vi "Configure Timebase Mode.vi"(6 "Window Range (5.0E-6)":dbl=5e-06, 8 "error in (no error)":errorcluster, 9 "Window Position (0.0 s)":dbl, 10 "Timebase Mode (0: Main)":u16(ring) items=["Main", "Window", "XY", "Roll"], 11 "VISA resource name":refnum<visa-resource-name>) -> (0 "error out":errorcluster, 3 "VISA resource name out":refnum<visa-resource-name>)   [LabVIEW 2017, in "Agilent 6000 Series.lvlib"]
doc: "This VI selects time base mode.\n\n<B>NOTE:</B>\n\nThe Window Timebase and Window Range controls are only valid when Timebase Mode is set to \"Window\"."
uses:
  <instrlib>/Agilent 6000 Series/Agilent 6000 Series.lvlib
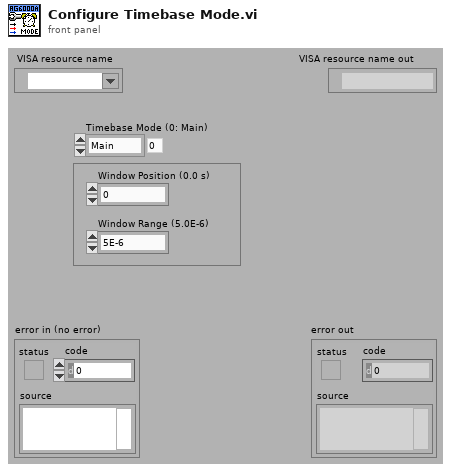
[diagram p1: front panel]
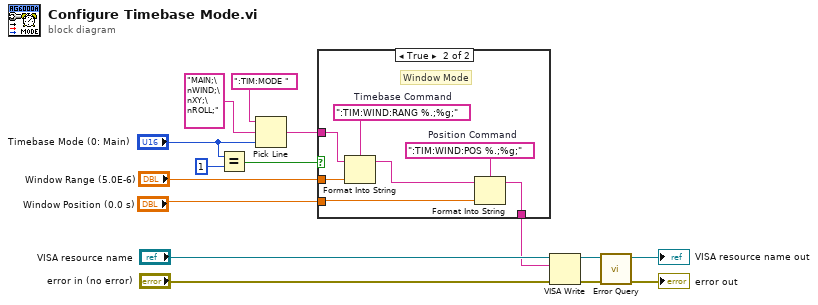
[diagram p0: block diagram]
diagram:
  n1 = Equal?(x="Timebase Mode (0: Main)", y=u16 1) -> (x = y?=w3:bool)
  n2 = Pick Line(string ("")=":TIM:MODE ", multi-line string="MAIN;\nWIND;\nXY;\nROLL;", line index="Timebase Mode (0: Main)") -> (output string=w4:string)
  n3 = case shown="True" w3 {
    tunnel: "Window Position (0.0 s)" -> [_ w20]
    tunnel: "Window Range (5.0E-6)" -> [_ w19]
    tunnel: [w16 w18] -> w5
    tunnel: w4 -> [w16 w17]
    frame False {
      # "Don't send commands\nif Mode isn't Window"
    }
    frame True {
      w22 = ":TIM:WIND:POS %.;%g;"  # Position Command
      w23 = ":TIM:WIND:RANG %.;%g;"  # Timebase Command
      # "Window Mode"
      n4 = Format Into String(format string=w23, initial string=w17, w19) -> (resulting string=w21:string)  [unwired: 1 in, 1 out]
      n5 = Format Into String(format string=w22, initial string=w21, w20) -> (resulting string=w18:string)  [unwired: 1 in, 1 out]
    }
  }
  n6 = VISA Write(VISA resource name="VISA resource name", write buffer=w5, error in (no error)="error in (no error)") -> (VISA resource name out=w11:refnum<visa-resource-name>, error out=w10:errorcluster)  [unwired: 1 out]
  n7 = call <instrlib>:"Error Query.vi"("error in (no error)"=w10, "VISA resource name"=w11) -> ("error out"=→"error out":errorcluster, "VISA resource name out"=→"VISA resource name out":refnum<visa-resource-name>)  [unwired: 6 in, 2 out]
